vi "Status Get Pressure.vi"(5 "Retry Attempts (0)":i32 min=0, 8 "error in":errorcluster, 11 "VISA resource name":refnum<visa-resource-name>) -> (0 "error out":errorcluster, 2 "Pressure":i32, 3 "VISA resource name out":refnum<visa-resource-name>)   [LabVIEW 2020, in "ChromTech Series III Pump.lvlib"]
doc: "Query the pump for the current pressure value."
uses:
  <instrlib>/RxnRover/ChromtechSeriesIIIDriver/ChromTech Series III Pump.lvlib
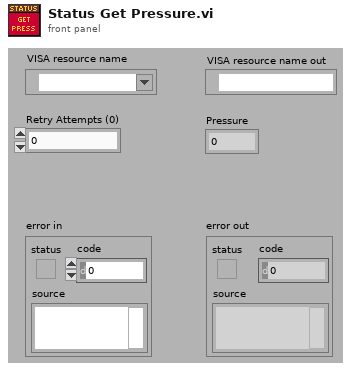
[diagram p1: front panel]
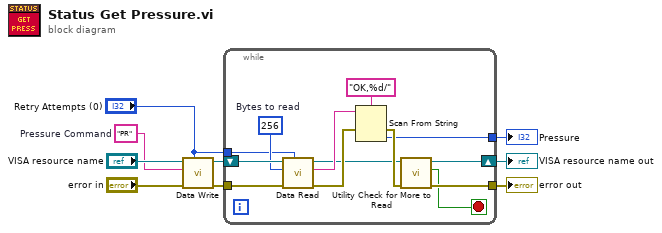
[diagram p0: block diagram]
diagram:
  w4 = "PR"  # Pressure Command
  n1 = call <instrlib>:"Data Write.vi"("Retry Attempts (0)"="Retry Attempts (0)", "error in (no error)"="error in", "Command"=w4, "VISA Refnum in"="VISA resource name") -> ("error out"=w5:errorcluster, "VISA Refnum out"=w8:refnum<visa-resource-name>)  [unwired: 6 in]
  n2 = while {
    tunnel: [w17] -> w2
    tunnel: "Retry Attempts (0)" -> [w14]
    shift-right: [w11] -> w7
    shift-left: w8 -> [w22]
    tunnel: w5 -> [w21]
    tunnel: [w13] -> w3
    stop <- w10 stop-if-true
    w20 = u32 256  # Bytes to read
    n3 = call <instrlib>:"Data Read.vi"("Retry Attempts (0)"=w14, "error in (no error)"=w21, "Bytes to read"=w20, "VISA Refnum in"=w22) -> ("error out"=w19:errorcluster, "read buffer"=w16:string, "VISA Refnum out"=w12:refnum<visa-resource-name>)  [unwired: 5 in]
    n4 = Scan From String(format string="OK,%d/", input string=w16, error in=w19) -> (error out=w18:errorcluster, output 1=w17:i32)  [unwired: 2 in, 2 out]
    n5 = call <instrlib>:"Utility Check for More to Read.vi"("error in (no error)"=w18, "VISA Refnum in"=w12) -> ("error out (unchanged)"=w13:errorcluster, "More to read?"=w10:bool, "VISA Refnum out"=w11:refnum<visa-resource-name>)  [unwired: 7 in]
  }
  "VISA resource name out" <- w7
  "error out" <- w3
  "Pressure" <- w2
